vi "Im the Bearer.vi"(8 "error in (no error)":errorcluster, 11 "Guardian in":refnum<class "Guardian.lvclass">) -> (0 "error out":errorcluster, 2 "I'm the Bearer":bool, 3 "Guardian out":refnum<class "Guardian.lvclass">)   [LabVIEW 2026, in "TALOS.lvlib" / "Guardian.lvlib" / "Guardian.lvclass"]
uses:
  Guardian.lvclass
  C:/LabVIEW Code/TALOS/talos/Ancestor/Ancestor/Ancestor.lvclass
  Ancestor/Ancestor/Ancestor.lvclass/Ancestor.ctl
  Guardian.lvclass/Guardian.ctl
  Ancestor/Ancestor/Ancestor.lvclass
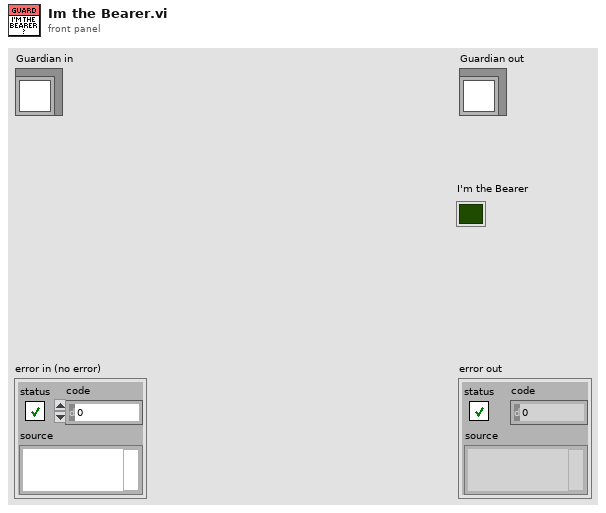
[diagram p1: front panel]
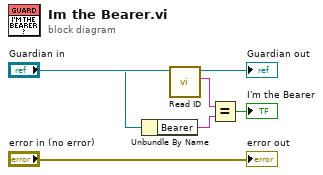
[diagram p0: block diagram]
diagram:
  n1 = call "Read ID.vi"("Ancestor in"="Guardian in") -> ("ID"=w3:string, "Ancestor out"=w4:refnum<class "Guardian.lvclass">)  [unwired: 8 in, 1 out]
  "Guardian out" <- w4
  n2 = Unbundle By Name(w4) -> ("Bearer"=w2:string)
  n3 = Equal?(x=w3, y=w2) -> (x = y?=→"I'm the Bearer":bool)
  "error out" <- "error in (no error)"
